vi "20151109 NN scaling.vi"(10 "Input":dbl[](array[numeric]), 11 "Neural Network Out":T1) -> (3 "Output":dbl[](array[numeric]))   [LabVIEW 2013]
uses:
  SSNN(super simple neural network)_2.1/Neural Network/Types/Neural Network.ctl
  SSNN(super simple neural network)_2.1/Neural Network/Types/2D Array.ctl
  SSNN(super simple neural network)_2.1/Neural Network/Types/Scaling Info.ctl
  <vilib>/Analysis/NI_AALBase.lvlib
  SSNN(super simple neural network)_2.1/Neural Network/Super Simple Neural Network.lvlib
panel:
  in  "Method":enum16{"No scale", "Scale 0", "Scale 1"}(ring)=enum."Scale 0"
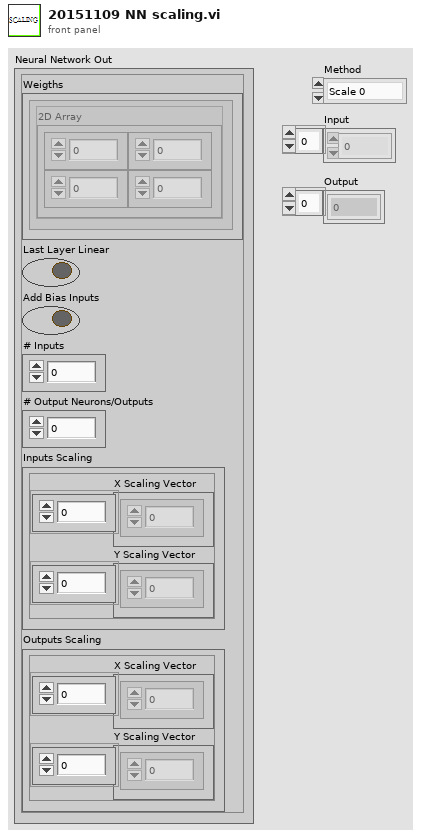
[diagram p1: front panel]
types:
  T1 = typedef "Super Simple Neural Network.lvlib/Neural Network.ctl" = cluster{"Weigths":T2[], "Last Layer Linear":bool, "Add Bias Inputs":bool, "# Inputs":u32, "# Output Neurons/Outputs":u32, "Inputs Scaling":T3, "Outputs Scaling":T3}
  T2 = typedef "Super Simple Neural Network.lvlib/2D Array.ctl" = cluster{"2D Array":dbl[][]}
  T3 = typedef "Super Simple Neural Network.lvlib/Scaling Info.ctl" = cluster{"X Scaling Vector":dbl[], "Y Scaling Vector":dbl[]}
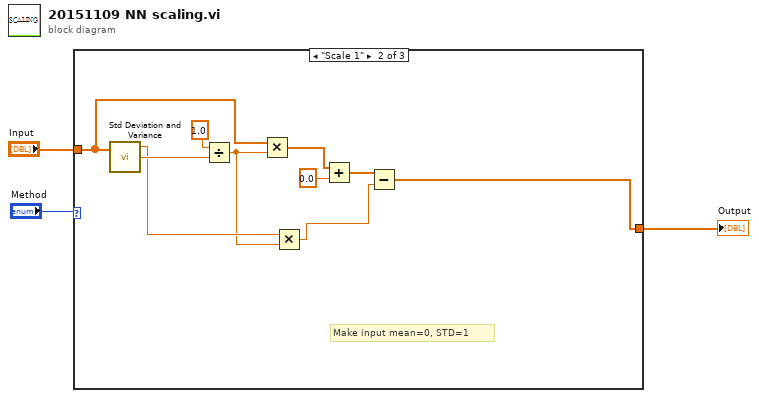
[diagram p0: block diagram]
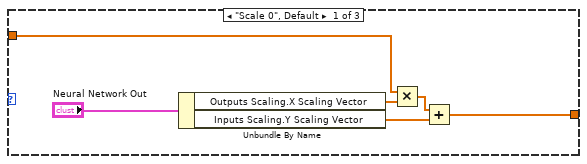
[diagram p2: hidden frame]
diagram:
  n1 = case shown="\"Scale 1\"" "Method" {
    tunnel: [w9 w10 w20] -> w3
    tunnel: "Input" -> [w4 w17 w20]
    frame "Scale 0", Default {
      n2 = Unbundle By Name("Neural Network Out") -> ("Outputs Scaling.X Scaling Vector"=w7:dbl[], "Inputs Scaling.Y Scaling Vector"=w8:dbl[])
      n3 = Multiply(x=w4, y=w7) -> (x*y=w6:dbl[])
      n4 = Add(x=w6, y=w8) -> (x+y=w9:dbl[])
    }
    frame "Scale 1" {
      # "Make input mean=0, STD=1"
      n5 = call <vilib>:"Std Deviation and Variance.vi"("X"=w17) -> ("mean"=w13:dbl, "standard deviation"=w19:dbl)  [unwired: 1 in, 1 out]
      n6 = Divide(x=1.0, y=w19) -> (x/y=w12:dbl)
      n7 = Multiply(x=w17, y=w12) -> (x*y=w16:dbl[])
      n8 = Multiply(x=w13, y=w12) -> (x*y=w11:dbl)
      n9 = Add(x=w16, y=0.0 ("x")) -> (x+y=w14:dbl[])
      n10 = Subtract(x=w14, y=w11) -> (x-y=w10:dbl[])
    }
    frame "No scale" {
    }
  }
  "Output" <- w3
